vi "DrawDialog.vi"(8 "error in (no error)":errorcluster, 10 "RT_Game.lvlib:Game.lvclass":refnum<class "Game.lvclass">, 11 "Highscore in":refnum<class "HighscoreDialog.lvclass">) -> (0 "error out":errorcluster, 2 "GameOut":refnum<class "Game.lvclass">, 3 "Highscore out":refnum<class "HighscoreDialog.lvclass">)   [LabVIEW 2019, in "RT_Game.lvlib" / "HighscoreDialog.lvclass"]
uses:
  HighscoreDialog/HighscoreDialog.lvclass
  C:/Users/FreshBob/Dropbox/VIs/myRIO_GameConsole/RT/RT_Game/GameObject/GameObject.lvclass
  Game/Game.lvclass
  Game/Coordinate.ctl
  GameObject/GameObject.lvclass/GameObject.ctl
  HighscoreDialog/HighscoreDialog.lvclass/HighscoreDialog.ctl
  GameObject/Read position.vi
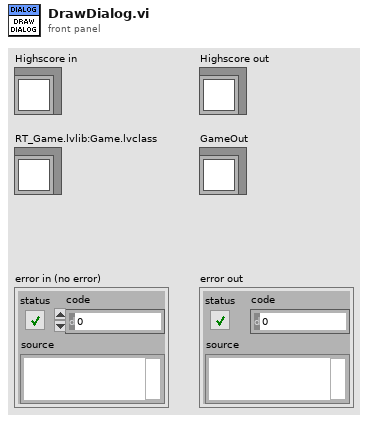
[diagram p1: front panel]
types:
  T1 = typedef "RT_Game.lvlib/Game.lvclass/Coordinate.ctl" = cluster{"x":dbl, "y":dbl}
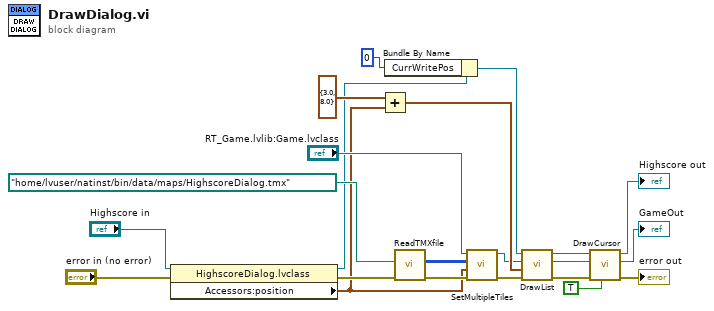
[diagram p0: block diagram]
diagram:
  n1 = property class="HighscoreDialog.lvclass"(reference="Highscore in", error in="error in (no error)") -> (reference out=w4:refnum<class "HighscoreDialog.lvclass">, error out=w6:errorcluster, "Accessors:position"=w1:T1)
  n2 = Add(x=T1 {"x"=3.0, "y"=8.0} ("y"), y=w1) -> (x+y=w19:T1)
  n3 = Bundle By Name(cluster=w4, "CurrWritePos"=i16 0 ("CurrPos")) -> (w3:refnum<class "HighscoreDialog.lvclass">)
  n4 = call "ReadTMXfile.vi"("error in (no error)"=w6, "path to tmx-file (created with Tiles2D)"=path "/home/lvuser/natinst/bin/data/maps/HighscoreDialog.tmx") -> ("error out"=w9:errorcluster, "Tilenumbers"=w14:u32[][])  [unwired: 8 in]
  n5 = call "SetMultipleTiles.vi"("error in (no error)"=w9, "Position"=w1, "TileCodes"=w14, "Game in"="RT_Game.lvlib:Game.lvclass") -> ("error out"=w15:errorcluster, "Game out"=w17:refnum<class "Game.lvclass">)  [unwired: 6 in]
  n6 = call "DrawList.vi"("error in (no error)"=w15, "Position"=w19, "GameIn"=w17, "Highscore in"=w3) -> ("error out"=w16:errorcluster, "GameOut"=w21:refnum<class "Game.lvclass">, "Highscore out"=w20:refnum<class "HighscoreDialog.lvclass">)  [unwired: 5 in]
  n7 = call "DrawCursor.vi"("Visible?"=TRUE, "error in (no error)"=w16, "GameIn"=w21, "Highscore in"=w20) -> ("error out"=→"error out":errorcluster, "GameOut"=→"GameOut":refnum<class "Game.lvclass">, "Highscore out"=→"Highscore out":refnum<class "HighscoreDialog.lvclass">)  [unwired: 5 in]
